vi "DHE_SetReadMode.vi"(0 "refnum":i32=2048, 7 "readmode":string, 11 "error in (no error)":errorcluster) -> (4 "fd out":i32, 6 "return value":i32, 8 "X total size":u16, 10 "Y total size":u16, 14 "DET_READ_TIME":sgl=3.5 format="%.2f", 15 "error out":errorcluster)   [LabVIEW 2016]
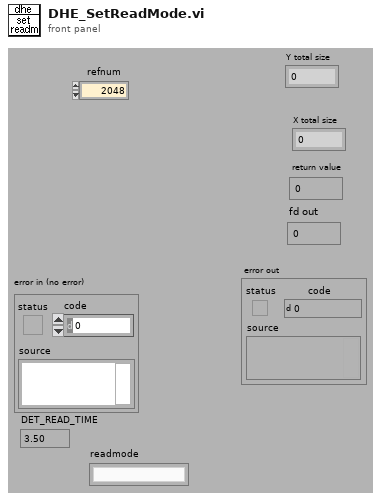
[diagram p1: front panel]
types:
  T1 = typedef "GEOM_CorrectedFPA.ctl" = cluster{"readmode":string, "amplifiers":cluster{"number":i32, "xstart":i32, "ystart":i32}[], "totxsize":i32, "totysize":i32, "maxxdim":i32, "maxydim":i32, "numxamps":i32, "numyamps":i32, "totxdata":i32, "totydata":i32, "xdataamp":i32, "ydataamp":i32, "totpixels":i32}
  T2 = typedef "GEOM_Amplifier.ctl" = cluster{"number":i32, "type":T3, "rotated":i16, "fliped":u16, "FPAcoord":cluster{"xstart":i32, "ystart":i32}, "Physical_size":cluster{"columns":i32, "rows":i32}, "predata":cluster{"columns":i32, "rows":i32}, "postdata":cluster{"columns":i32, "rows":i32}, "Req ROIs":T4, "Corr ROI":T4, "Detnumber":i32, "ampID":string, "discard":i32}
  T3 = typedef "GEOM_AmpType.ctl" = u16
  T4 = typedef "GEOM_ROI.ctl" = T5[]
  T5 = typedef "GEOM_Coords.ctl" = cluster{"xstart":u32, "ystart":u32, "xsize":u32, "ysize":u32}
  T6 = typedef "DatabaseHand_RefNum.ctl" = refnum<vi>
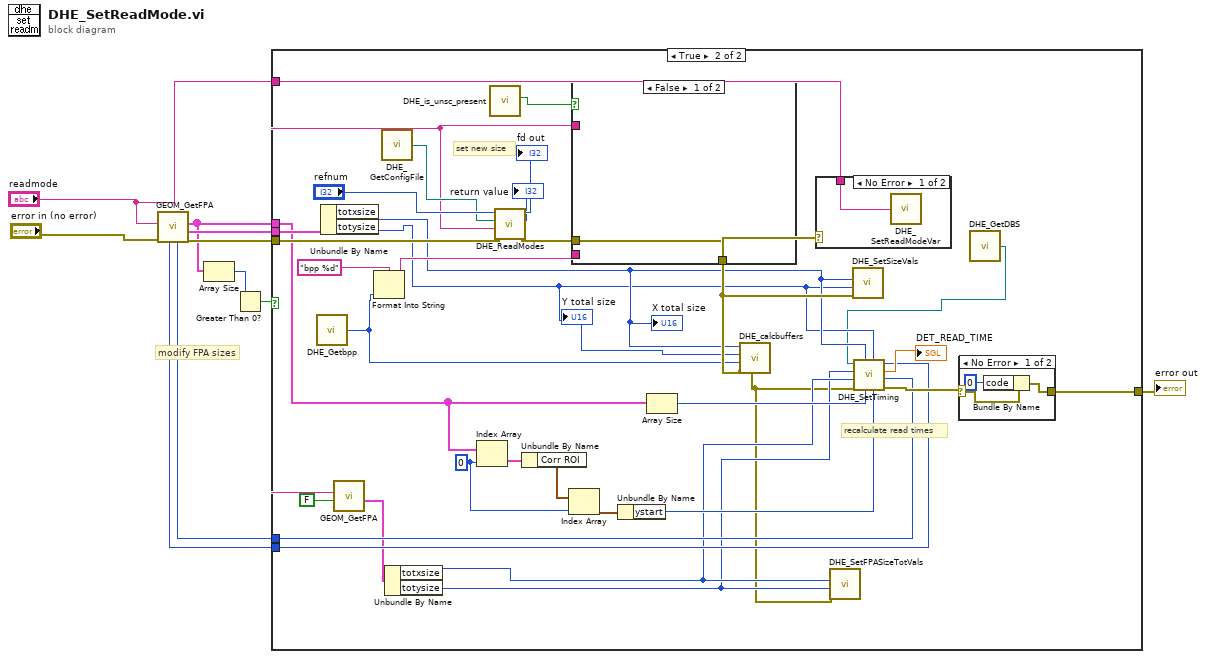
[diagram p0: block diagram]
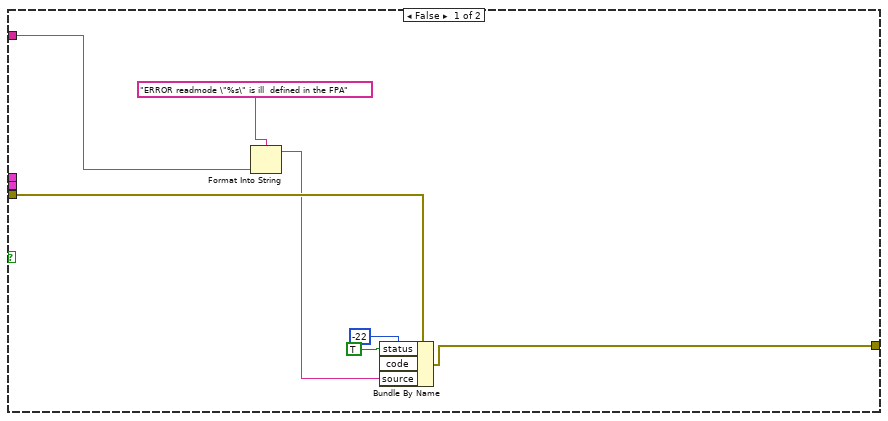
[diagram p2: hidden frame]
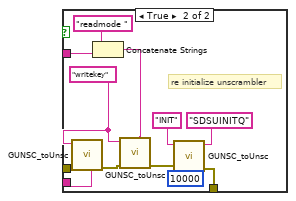
[diagram p3: hidden frame]
diagram:
  # "modify FPA sizes"
  n1 = call "GEOM_GetFPA.vi"("error in (no error)"="error in (no error)", "readmode"="readmode") -> ("error out"=w10:errorcluster, "CorrectedFPACoord"=w9:T1, "amplifiers"=w3:T2[], "numyamps"=w5:i32, "numxamps"=w6:i32)  [unwired: 1 in, 4 out]
  n2 = Array Size(array=w3) -> (size(s)=w2:i32)
  n3 = Greater Than 0?(x=w2) -> (x > 0?=w1:bool)
  n4 = case shown="True" w1 {
    tunnel: w10 -> [w17 w49]
    tunnel: w9 -> [_ w48]
    tunnel: [w16 w42] -> w7
    tunnel: w6 -> [_ w30]
    tunnel: w5 -> [_ w29]
    tunnel: "readmode" -> [w12 w18]
    tunnel: w3 -> [_ w20]
    frame False {
      n5 = Format Into String(format string="ERROR readmode \"%s\" is ill  defined in the FPA" ("source"), w12) -> (resulting string=w11:string)  [unwired: 2 in, 1 out]
      n6 = Bundle By Name(cluster=w17, "status"=TRUE, "code"=-22, "source"=w11) -> (w16:errorcluster)
    }
    frame True {
      w33 = 0 ("index")
      # "recalculate read times"
      # "set new size"
      n7 = call "DHE_Getbpp.vi"() -> ("DHE_bpp"=w22:i32)  [unwired: 9 out]
      n8 = Unbundle By Name(w48) -> ("totxsize"=w37:i32, "totysize"=w36:i32)
      "Y total size" <- w36
      "X total size" <- w37
      n9 = call "GEOM_GetFPA.vi"("binned?"=FALSE, "readmode"=w18) -> ("CorrectedFPACoord"=w27:T1)  [unwired: 1 in, 8 out]
      n10 = Format Into String(format string="bpp %d", w22) -> (resulting string=w40:string)  [unwired: 2 in, 1 out]
      n11 = call "DHE_GetConfigFile.vi"() -> ("DHE_ConfigFile"=w23:path)  [unwired: 9 out]
      n12 = Unbundle By Name(w27) -> ("totxsize"=w26:i32, "totysize"=w25:i32)
      n13 = Index Array(array=w20, index=w33) -> (element=w35:T2)
      n14 = call "DHE_is_unsc_present.vi"() -> ("value"=w21:bool)  [unwired: 1 in, 10 out]
      n15 = call "DHE_ReadModes.vi"("error in (no error)"=w49, "read mode"=w18, "configuration file path"=w23, "fd"="refnum") -> ("error out"=w41:errorcluster, "error_code"=→"return value":i32, "fd out"=→"fd out":i32)  [unwired: 5 out]
      n16 = Unbundle By Name(w35) -> ("Corr ROI"=w34:T4)
      n17 = Index Array(array=w34, index=w33) -> (element=w32:T5)
      n18 = case shown="False" w21 {
        tunnel: [w51 w57] -> w44
        tunnel: w41 -> [w51 w56]
        tunnel: w40 -> [_ w53]
        tunnel: w18 -> [_ w52]
        frame False {
        }
        frame True {
          w54 = "writekey" ("command")
          # "re initialize unscrambler"
          n19 = call "GUNSC_toUnsc.vi"("key"=w53, "error in (no error)"=w56, "command"=w54) -> ("error out"=w55:errorcluster)  [unwired: 6 in, 2 out]
          n20 = Concatenate Strings("readmode " ("string"), w52) -> (w59:string)
          n21 = call "GUNSC_toUnsc.vi"("key"=w59, "error in (no error)"=w55, "command"=w54) -> ("error out"=w60:errorcluster)  [unwired: 6 in, 2 out]
          n22 = call "GUNSC_toUnsc.vi"("responseQ"="SDSUINITQ", "bpp"=10000 ("ms timeout (-1)"), "error in (no error)"=w60, "command"="INIT") -> ("error out"=w57:errorcluster)  [unwired: 5 in, 2 out]
        }
      }
      n23 = Unbundle By Name(w32) -> ("ystart"=w31:u32)
      n24 = Array Size(array=w20) -> (size(s)=w39:i32)
      n25 = call "DHE_calcbuffers.vi"("error in (no error)"=w44, "bpp"=w22, "nrows"=w36, "ncols"=w37) -> ("error out"=w24:errorcluster)  [unwired: 2 in, 5 out]
      n26 = case shown="No Error" w44 {
        tunnel: w18 -> [w68 _]
        frame No Error {
          n27 = call "DHE_SetReadModeVar.vi"("DHE_ReadMode"=w68) -> ()  [unwired: 9 out]
        }
        frame Error {
        }
      }
      n28 = call "DHE_SetFPASizeTotVals.vi"("error in"=w24, "ytotsize"=w25, "xtotsize"=w26) -> ()  [unwired: 9 out]
      n29 = call "DHE_SetSizeVals.vi"("error in"=w44, "ytotsize"=w36, "xtotsize"=w37) -> ()  [unwired: 9 out]
      n30 = call "DHE_GetDBS.vi"() -> ("DHE_DBSRef"=w19:T6)  [unwired: 9 out]
      n31 = call "DHE_SetTiming.vi"("num of Y amps"=w29, "num of X amps"=w30, "yroi start"=w31, "roi rows"=w36, "Num of amps"=w39, "roi cols"=w37, "error in"=w24, "totysize"=w26, "totxsize"=w25, "Database RefNum out"=w19) -> ("errorout"=w43:errorcluster, "DET_READ_TIME"=→"DET_READ_TIME":sgl)
      n32 = case shown="No Error" w43 {
        selector: w43 -> [w66 w67]
        tunnel: [w64 w67] -> w42
        frame No Error {
          n33 = Bundle By Name(cluster=w66, "code"=0) -> (w64:errorcluster)
        }
        frame Error {
        }
      }
    }
  }
  "error out" <- w7
